vi "Basic RS232 Write Read.vi"() -> ()   [LabVIEW 2018, in "Support Library.lvlib"]
uses:
  Support Library.lvlib
  <vilib>/Instr/_visa.llb/VISA Configure Serial Port (Instr).vi
panel:
  out "read string":string
  out "VISA resource name Out":refnum<visa-resource-name>
  in  "VISA resource name In":refnum<visa-resource-name>
  out "error out":errorcluster
  in  "error in (no error)":errorcluster
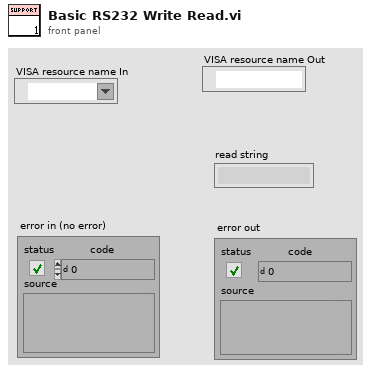
[diagram p1: front panel]
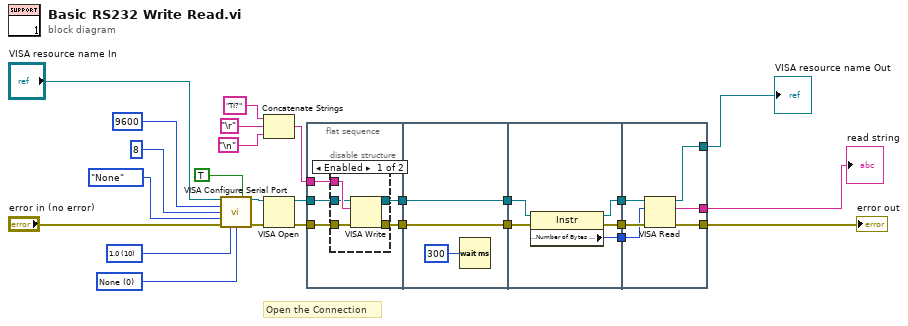
[diagram p0: block diagram]
diagram:
  w19 = u16 0 items=["None", "XON/XOFF", "RTS/CTS", "XON/XOFF & RTS/CTS", "DTR/DSR", "XON/XOFF & DTR/DSR"] ("flow control (0:none)")
  w20 = u16 10 items=["1.0"=10, "1.5"=15, "2.0"=20] ("stop bits (10: 1 bit)")
  # "Open the Connection"
  n1 = call-poly "VISA Configure Serial Port"("VISA resource name"="VISA resource name In", "Enable Termination\nChar (T)"=TRUE ("Enable Termination\nChar (T)"), "baud rate (9600)"=u32 9600, "data bits (8)"=u16 8, "parity (0:none)"=enum16{"None", "Odd", "Even", "Mark", "Space"}."None", "error in (no error)"="error in (no error)", "stop bits (10: 1 bit)"=w20, "flow control (0:none)"=w19) -> ("VISA resource name out"=w17:refnum<visa-resource-name>, "error out"=w18:errorcluster)  [unwired: 6 in]
  n2 = Concatenate Strings("TI?", "\r", "\n") -> (w14:string)
  n3 = VISA Open(error in (no error)=w18, VISA resource name=w17) -> (VISA resource name=w25:refnum<visa-resource-name>, error out=w15:errorcluster)  [unwired: 3 in]
  n4 = flat-sequence {
    tunnel: w14 -> [w31]
    tunnel: [w30] -> w9
    tunnel: [w29] -> w8
    tunnel: w25 -> [w28]
    tunnel: w15 -> [w27]
    tunnel: w9 -> [w40]
    tunnel: w8 -> [w39]
    tunnel: [w40] -> w7
    tunnel: [w39] -> w6
    tunnel: [w44] -> w5
    tunnel: [w43] -> w4
    tunnel: [w42] -> w3
    tunnel: w7 -> [w46]
    tunnel: w6 -> [w45]
    tunnel: [w52] -> w10
    tunnel: [w51] -> w11
    tunnel: [w50] -> w12
    tunnel: w5 -> [w49]
    tunnel: w4 -> [w48]
    tunnel: w3 -> [w47]
    frame #0 {
      n5 = disable-structure shown="Enabled" {
        disable-tunnel: w31 -> [w36 _]
        disable-tunnel: [w35 w38] -> w30
        disable-tunnel: [w34 w37] -> w29
        disable-tunnel: w28 -> [w33 w38]
        disable-tunnel: w27 -> [w32 w37]
        frame Enabled {
          n6 = VISA Write(VISA resource name=w33, write buffer=w36, error in (no error)=w32) -> (VISA resource name out=w35:refnum<visa-resource-name>, error out=w34:errorcluster)  [unwired: 1 out]
        }
        frame Disabled {
        }
      }
    }
    frame #1 {
      n7 = Wait (ms)(milliseconds to wait=u32 300) -> ()  [unwired: 1 out]
    }
    frame #2 {
      n8 = property class="Instr"(reference=w46, error in=w45) -> (reference out=w44:refnum<visa-resource-name>, error out=w43:errorcluster, "Serial Settings:Number of Bytes at Serial Port"=w42:u32)
    }
    frame #3 {
      n9 = VISA Read(VISA resource name=w49, byte count=w47, error in (no error)=w48) -> (VISA resource name out=w50:refnum<visa-resource-name>, read buffer=w51:string, error out=w52:errorcluster)  [unwired: 1 out]
    }
  }
  "error out" <- w10
  "VISA resource name Out" <- w12
  "read string" <- w11
